vi "CenterOneDriverServer.vi"   [LabVIEW 2010, in "CenterOne.lvlib"]
uses:
  CenterOne.lvlib
  Comunication Status.ctl
types:
  T1 = typedef "CenterOne.lvlib/Comunication Status.ctl" = string
  T2 = typedef "CenterOne.lvlib/Serial Config.ctl" = cluster{"串口选择":refnum<visa-resource-name>, "通讯速率":u32, "超时时间":u32, "数据位长":u16, "奇偶校验":enum16{"None", "Odd", "Even", "Mark", "Space"}, "停止位长":u16, "握手控制":u16, "字符结束":bool, "结束字符":u8}
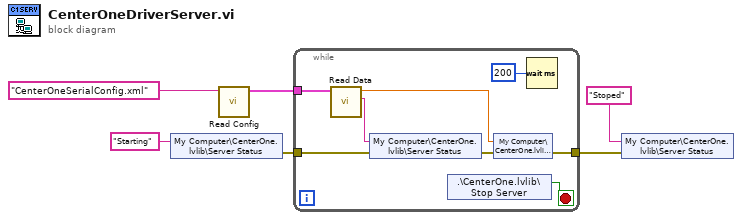
[diagram p0: block diagram]
diagram:
  n1 = shared-variable "My Computer\\CenterOne.lvlib\\Server Status"(T1 "Starting" ("Server Status")) -> (error out=w5:errorcluster)  [unwired: 1 in]
  n2 = call "Read Config.vi"("FileName"="CenterOneSerialConfig.xml") -> ("Serial Config"=w1:T2)  [unwired: 9 in, 1 out]
  n3 = while {
    tunnel: [w7] -> w6
    tunnel: w5 -> [w9]
    tunnel: w1 -> [w12]
    stop <- w13 stop-if-true
    n4 = call "Read Data.vi"("Serial Config"=w12) -> ("状态信息"=w10:string, "返回值"=w11:dbl)  [unwired: 8 in, 1 out]
    n5 = shared-variable "My Computer\\CenterOne.lvlib\\Server Status"(w10, error in=w9) -> (error out=w8:errorcluster)
    n6 = shared-variable ".\\CenterOne.lvlib\\Stop Server"() -> (w13:bool)  [unwired: 1 in, 1 out]
    n7 = shared-variable "My Computer\\CenterOne.lvlib\\RV"(w11, error in=w8) -> (error out=w7:errorcluster)
    n8 = Wait (ms)(milliseconds to wait=u32 200) -> ()  [unwired: 1 out]
  }
  n9 = shared-variable "My Computer\\CenterOne.lvlib\\Server Status"(T1 "Stoped" ("Server Status"), error in=w6) -> ()  [unwired: 1 out]
